vi "GetType.vi"(8 "error in (no error)":errorcluster, 11 "Configure Scaling Msg":refnum<class "Configure Scaling Msg.lvclass">) -> (0 "error out":errorcluster, 2 "Data Sample":variant, 3 "Configure Scaling Msg":refnum<class "Configure Scaling Msg.lvclass">)   [LabVIEW 2015, in "CS++Motor.lvlib" / "Configure Scaling Msg.lvclass"]
uses:
  Configure Scaling Msg.lvclass
  Configure Scaling Msg.lvclass/Configure Scaling Msg.ctl
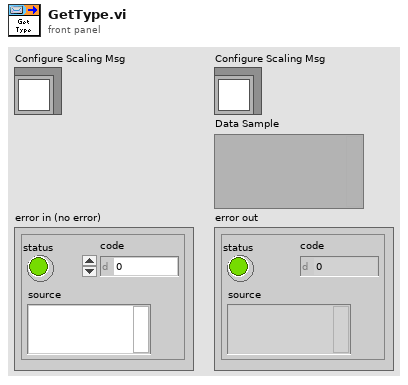
[diagram p1: front panel]
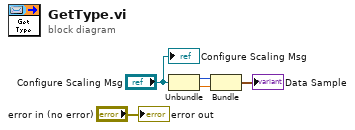
[diagram p0: block diagram]
diagram:
  n1 = Unbundle("Configure Scaling Msg") -> (w2:u8, w1:dbl)
  n2 = Bundle("AxisNumber"=w2, "Scaling"=w1) -> (→"Data Sample":cluster{"AxisNumber":u8, "Scaling":dbl})  [unwired: 1 in]
  "error out" <- "error in (no error)"
  "Configure Scaling Msg" <- "Configure Scaling Msg"
